vi "set_stage_init (SubVI).vi"(0 "Tot Stage Arr":dbl[](array[numeric]), 5 "electrode arr":dbl[][](array[numeric]), 7 "flash_arr":dbl[](array[numeric]), 9 "electrodes task":refnum<k21>, 11 "electrodes task error":errorcluster) -> (4 "init_arr":dbl[][](array[numeric]), 10 "electrodes task 2":refnum<k21>, 15 "electrodes task error 2":errorcluster)   [LabVIEW 2018]
uses:
  <vilib>/DAQmx/write.llb/DAQmx Write (Analog 2D DBL NChan NSamp).vi
  <vilib>/DAQmx/miscellaneous.llb/DAQmx Fill In Error Info.vi
  <vilib>/measure/NI_MABase.lvlib
  <resource>/objmgr/daqmx.rc
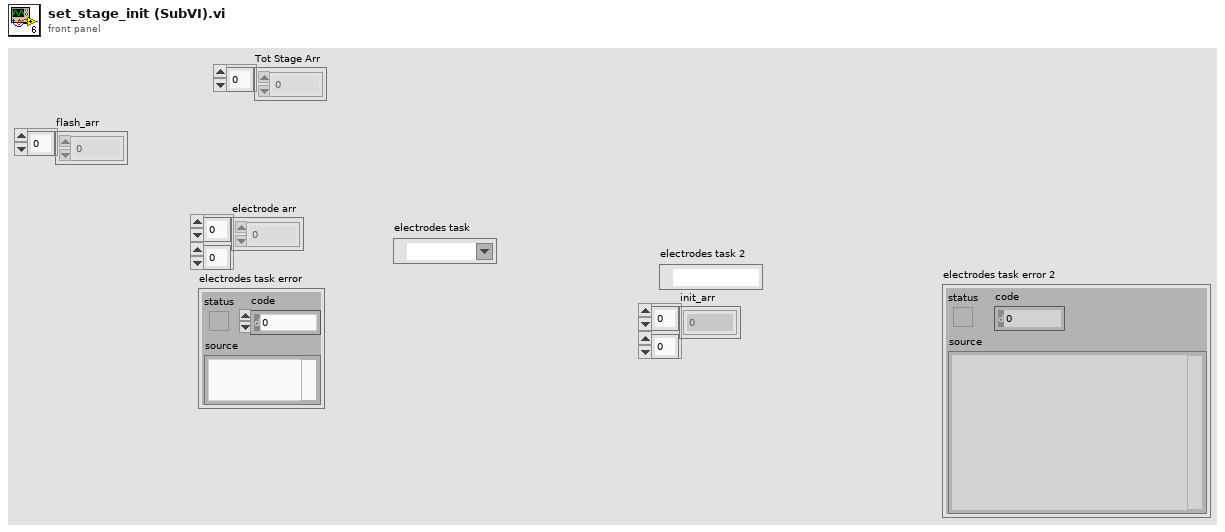
[diagram p1: front panel]
types:
  T1 = enum16{"Sine Wave", "Triangle Wave", "Square Wave", "Sawtooth Wave"}
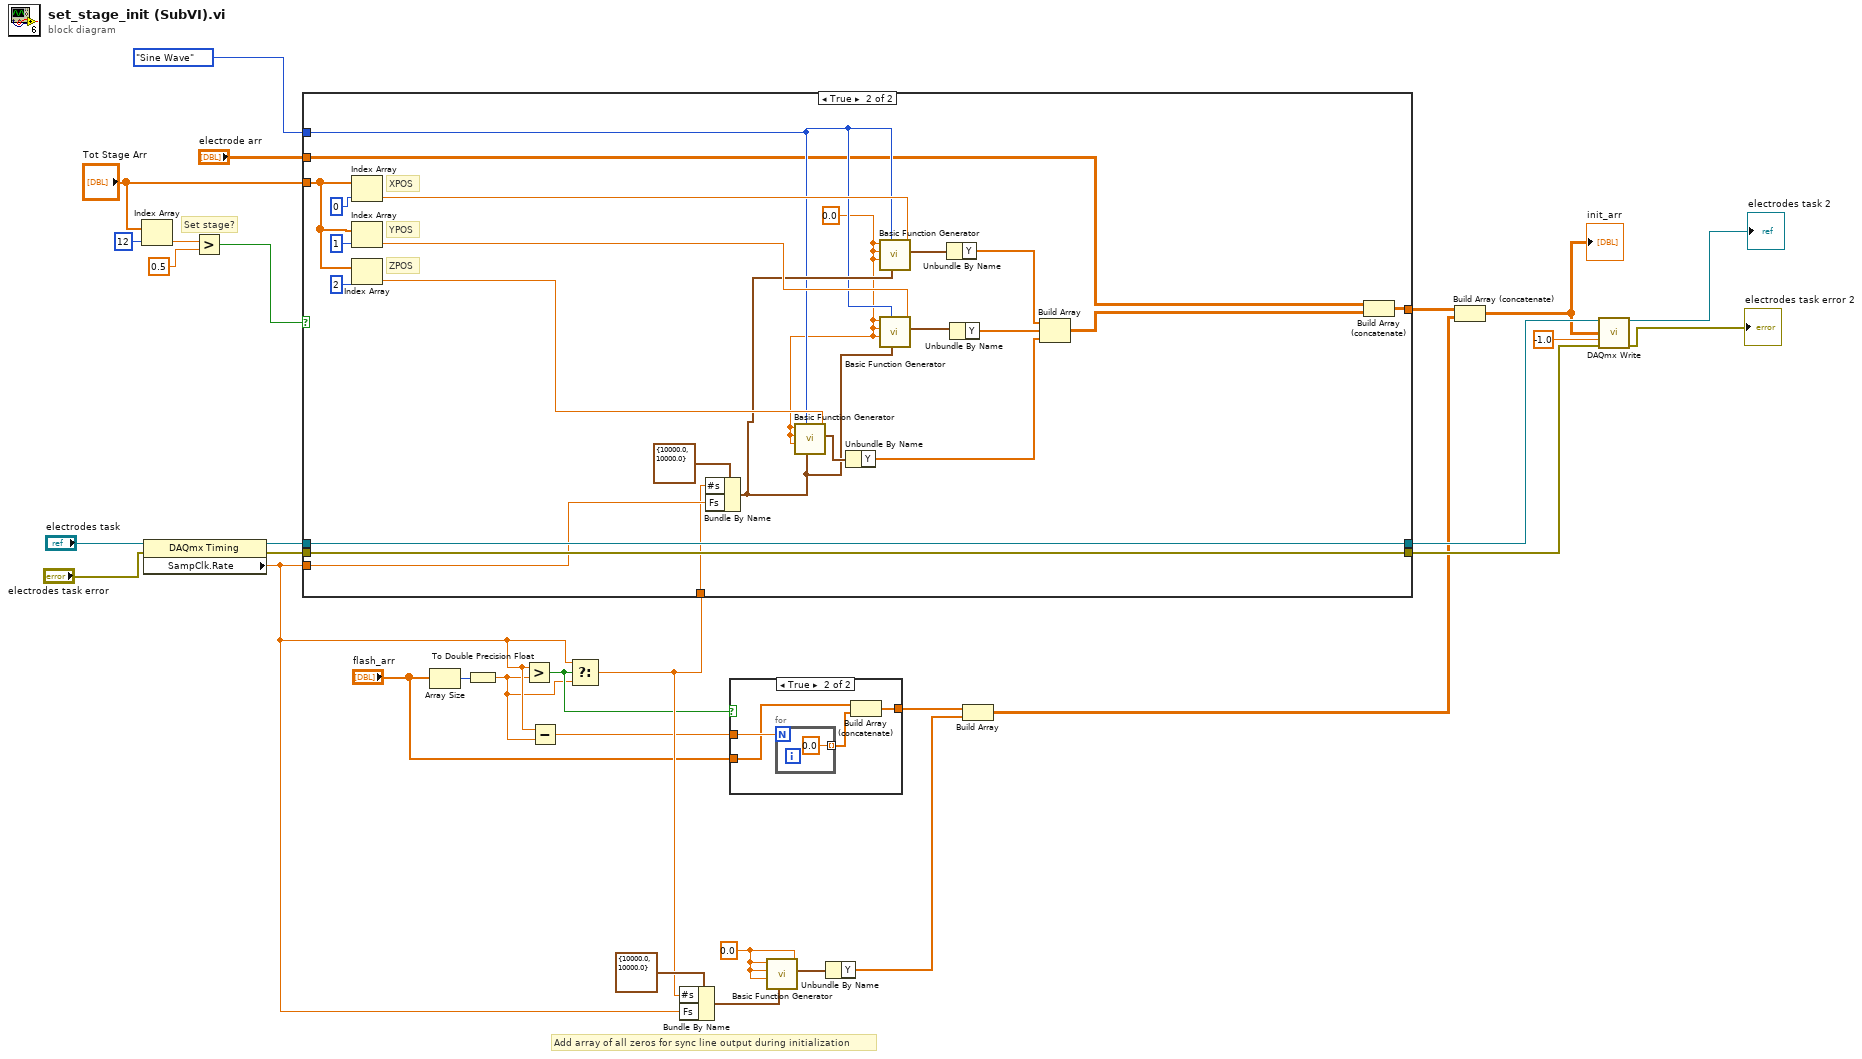
[diagram p0: block diagram]
diagram:
  w13 = 0.0 ("amplitude")
  # "Add array of all zeros for sync line output during initialization"
  # "Set stage?"
  n1 = Index Array(array="Tot Stage Arr", index=12) -> (element=w31:dbl)
  n2 = property class="DAQmx Timing"(reference="electrodes task", error in="electrodes task error") -> (reference out=w20:refnum<k21>, error out=w19:errorcluster, "SampClk.Rate"=w3:dbl)
  n3 = Greater?(x=w31, y=0.5) -> (0:w29:bool)
  n4 = Array Size(array="flash_arr") -> (size(s)=w10:i32)
  n5 = To Double Precision Float(number=w10) -> (double precision float=w2:dbl)
  n6 = Greater?(x=w3, y=w2) -> (0:w8:bool)
  n7 = Subtract(x=w3, y=w2) -> (x-y=w1:dbl)
  n8 = Select(t=w3, s=w8, f=w2) -> (s? t:f=w9:dbl)
  n9 = case shown="True" w29 {
    tunnel: "electrode arr" -> [w35 w41]
    tunnel: [w35 w56] -> w12
    tunnel: "Tot Stage Arr" -> [_ w49]
    tunnel: w20 -> [w34 w39]
    tunnel: w19 -> [w33 w38]
    tunnel: [w34 w39] -> w24
    tunnel: [w33 w38] -> w23
    tunnel: T1."Sine Wave" ("signal type") -> [_ w44]
    tunnel: w3 -> [_ w37]
    tunnel: w9 -> [_ w36]
    frame False {
    }
    frame True {
      w40 = 0.0 ("y")
      # "ZPOS"
      # "YPOS"
      # "XPOS"
      n10 = Index Array(array=w49, index=0) -> (element=w48:dbl)
      n11 = Index Array(array=w49, index=1) -> (element=w47:dbl)
      n12 = Index Array(array=w49, index=2) -> (element=w46:dbl)
      n13 = Bundle By Name(cluster=cluster{"Fs":dbl, "#s":dbl} {"Fs"=10000.0, "#s"=10000.0} ("sampling info"), "#s"=w36, "Fs"=w37) -> (w45:cluster{"Fs":dbl, "#s":dbl})
      n14 = call <vilib>:"Basic Function Generator.vi"("offset"=w46, "sampling info"=w45, "signal type"=w44, "phase"=w40, "amplitude"=w40, "frequency"=w40) -> ("signal out"=w53:waveform(dbl))  [unwired: 3 in, 2 out]
      n15 = Unbundle By Name(w53) -> ("Y"=w42:dbl[])
      n16 = call <vilib>:"Basic Function Generator.vi"("offset"=w48, "sampling info"=w45, "signal type"=w44, "phase"=w40, "amplitude"=w40, "frequency"=w40) -> ("signal out"=w54:waveform(dbl))  [unwired: 3 in, 2 out]
      n17 = call <vilib>:"Basic Function Generator.vi"("offset"=w47, "sampling info"=w45, "signal type"=w44, "phase"=w40, "amplitude"=w40, "frequency"=w40) -> ("signal out"=w55:waveform(dbl))  [unwired: 3 in, 2 out]
      n18 = Unbundle By Name(w54) -> ("Y"=w52:dbl[])
      n19 = Unbundle By Name(w55) -> ("Y"=w51:dbl[])
      n20 = Build Array(w52, w51, w42) -> (w50:dbl[][])
      n21 = Build Array (concatenate)(w41, w50) -> (w56:dbl[][])
    }
  }
  n22 = Bundle By Name(cluster=cluster{"Fs":dbl, "#s":dbl} {"Fs"=10000.0, "#s"=10000.0} ("sampling info"), "#s"=w9, "Fs"=w3) -> (w15:cluster{"Fs":dbl, "#s":dbl})
  n23 = case shown="True" w8 {
    tunnel: "flash_arr" -> [w60 w62]
    tunnel: [w60 w61] -> w6
    tunnel: w1 -> [_ w64]
    frame False {
    }
    frame True {
      n24 = for {
        N: w64 -> [_]
        tunnel: [0.0 ("amplitude")] -> w63 mode=indexing
      }
      n25 = Build Array (concatenate)(w62, w63) -> (w61:dbl[])
    }
  }
  n26 = call <vilib>:"Basic Function Generator.vi"("offset"=w13, "sampling info"=w15, "phase"=w13, "amplitude"=w13, "frequency"=w13) -> ("signal out"=w14:waveform(dbl))  [unwired: 4 in, 2 out]
  n27 = Unbundle By Name(w14) -> ("Y"=w5:dbl[])
  n28 = Build Array(w6, w5) -> (w4:dbl[][])
  n29 = Build Array (concatenate)(w12, w4) -> (w11:dbl[][])
  "init_arr" <- w11
  n30 = call-poly <vilib>:"DAQmx Write.vi"("task/channels in"=w24, "data"=w11, "timeout"=-1.0, "error in"=w23) -> ("task out"=→"electrodes task 2":refnum<k21>, "error out"=→"electrodes task error 2":errorcluster)  [unwired: 9 in, 1 out]
